vi "Write Startup Run Headless Msg.vi"(10 "Startup Run Headless Msg":refnum<class "Run Headless Msg.lvclass">, 11 "RootModel in":refnum<class "RootModel.lvclass">) -> (3 "RootModel out":refnum<class "RootModel.lvclass">)   [LabVIEW 2019, in "RootModel.lvlib" / "RootModel.lvclass"]
uses:
  <vilib>/gpm_packages/@cs/mva-core/Source/RootModel/RootModel/RootModel.lvclass
  <vilib>/gpm_packages/@cs/mva-core/Source/RootModel/RootModel Messages/Run Headless Msg/Run Headless Msg.lvclass
  <vilib>/gpm_packages/@cs/mva-core/Source/RootModel/RootModel/RootModel.lvclass/RootModel.ctl
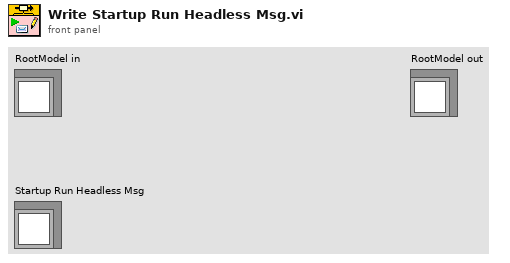
[diagram p1: front panel]
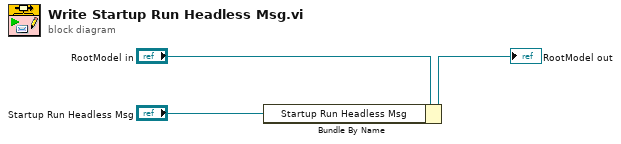
[diagram p0: block diagram]
diagram:
  n1 = Bundle By Name(cluster="RootModel in", "Startup Run Headless Msg"="Startup Run Headless Msg") -> (→"RootModel out":refnum<class "RootModel.lvclass">)
